vi "New.vi"() -> (0 "Root":refnum<class "Root.lvclass">)   [LabVIEW 2018, in "Toolkit.lvlib" / "Nodes.lvlib" / "Root.lvclass"]
doc: "Creates a new Abstract Syntax Tree (AST)."
uses:
  Root.lvclass
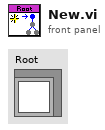
[diagram p1: front panel]
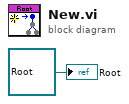
[diagram p0: block diagram]
diagram:
  "Root" <- refnum<class "Root.lvclass"> refnum ("Toolkit.lvlib:Nodes.lvlib:Root.lvclass")
